vi "Begin.vi"(8 "error in":errorcluster) -> (0 "error out":errorcluster)   [LabVIEW 2014]
doc: "Called before other user functions, this VI is expected to open initial I/O refnums, load in file data, and do all program initialization. Notice that the <B>error out</B> terminal is simply used for data flow. Wiring it to other structures or subVIs ensures that this VI runs first."
uses:
  <vilib>/Rock Robotics/WPI/SafetyOutput/WPI_SafetyOutputConfigMenu.ctl
  Robot Global Data.vi
  <vilib>/Rock Robotics/WPI/DriverStation/WPI_DriverStationRobotMode2.ctl
  <vilib>/Rock Robotics/WPI/Joystick/WPI_JoystickDeviceEnum.ctl
  <vilib>/Rock Robotics/SystemInterfaces/DIO/FPGA_DIOPWMChannel.ctl
  <vilib>/Rock Robotics/Network Tables/SD Write String Array.vi
  <vilib>/Rock Robotics/WPI/RobotDrive/WPI_RobotDriveOpen4MotorWithTalon.vi
  <vilib>/Rock Robotics/WPI/MotorControl/WPI_MotorControlOpen Talon.vi
  <vilib>/Rock Robotics/WPI/Counter/WPI_CounterDigitalInputToDigitalSource.vi
  <vilib>/Rock Robotics/SystemInterfaces/DIO/FPGA_DIOChannel.ctl
  <vilib>/Rock Robotics/Network Tables/SD Write Number.vi
  <vilib>/Rock Robotics/SystemInterfaces/AI/FPGA_AIGyroChannel.ctl
  <vilib>/Rock Robotics/SystemInterfaces/AI/FPGA_AIChannel.ctl
panel:
  # "t"
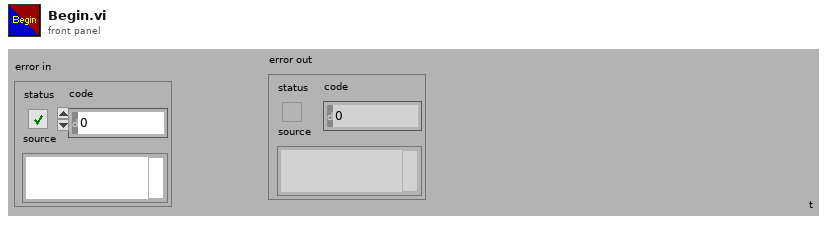
[diagram p1: front panel]
types:
  T1 = enum16{"Start", "Extending", "Lowering", "Grabbing", "Lifting", "Holding", "Placing", "Opening", "Dropping", "Score", "Exit", "Manual"}
  T2 = typedef "FPGA_DIOChannel.ctl" = enum8{"DIO 0", "DIO 1", "DIO 2", "DIO 3", "DIO 4", "DIO 5", "DIO 6", "DIO 7", "DIO 8", "DIO 9", "DIO MXP 0", "DIO MXP 1", "DIO MXP 2", "DIO MXP 3", "DIO MXP 4", "DIO MXP 5", "DIO MXP 6", "DIO MXP 7", "DIO MXP 8", "DIO MXP 9", "DIO MXP 10", "DIO MXP 11", "DIO MXP 12", "DIO MXP 13", "DIO MXP 14", "DIO MXP 15", "Invalid"}
  T3 = typedef "FPGA_AIChannel.ctl" = enum8{"AI 0", "AI 1", "AI 2", "AI 3", "AI MXP 0", "AI MXP 1", "AI MXP 2", "AI MXP 3", "Invalid"}
  T4 = typedef "FPGA_AIGyroChannel.ctl" = enum8{"AI 0", "AI 1", "Invalid"}
  T5 = typedef "FPGA_DIOPWMChannel.ctl" = enum8{"PWM 0", "PWM 1", "PWM 2", "PWM 3", "PWM 4", "PWM 5", "PWM 6", "PWM 7", "PWM 8", "PWM 9", "PWM MXP 0", "PWM MXP 1", "PWM MXP 2", "PWM MXP 3", "PWM MXP 4", "PWM MXP 5", "PWM MXP 6", "PWM MXP 7", "PWM MXP 8", "PWM MXP 9", "Invalid"}
  T6 = typedef "WPI_JoystickDeviceEnum.ctl" = enum16{"USB 0", "USB 1", "USB 2", "USB 3", "USB 4", "USB 5"}
  T7 = typedef "WPI_DriverStationRobotMode2.ctl" = enum16{"Autonomous Disabled", "Autonomous Enabled", "Teleop Disabled", "Teleop Enabled", "Disconnected", "Finish", "Test Disabled", "Test Enabled", "Emergency Stopped"}
  T8 = typedef "WPI_SafetyOutputConfigMenu.ctl" = enum16{"Enable", "Disable"}
  T9 = typedef "WPI_MotorControlDeviceRef.ctl" = cluster{"DeviceStatus":errorcluster, "Type":T10, "PWM":cluster{"Controller":T11, "PWM Channel":T5, "DeadBand":T12}, "CAN":cluster{"Device Number":u8, "Control Mode":T13, "Semaphore":T14, "Max Vout":dbl, "TalonSRX Control Mode":T15}, "Invert":bool, "TransformRef":T16, "InvTransformRef":T16}
  T10 = typedef "WPI_MotorControlType.ctl" = enum16{"PWM", "CAN", "CANTalonSRX"}
  T11 = typedef "FPGA_TypedefDigitalModule.ctl" = enum16{"Controller 1"}
  T12 = typedef "WPI_PWMDeadband.ctl" = cluster{"Name":string, "maxPositivePwm":i32, "minPositivePwm":i32, "centerPwm":i32, "maxNegativePwm":i32, "minNegativePwm":i32, "angularRange":u16}
  T13 = typedef "WPI_CANJaguar_ControlMode.ctl" = enum8{"Percent VBus", "Current", "Speed", "Position", "Voltage"}
  T14 = typedef "Semaphore RefNum" = refnum<k1>
  T15 = typedef "WPI_CANTalonSRX_APIControlMode.ctl" = enum8{"Percent VBus", "Speed", "Position", "Slave", "Unchanged / Invalid"}
  T16 = typedef "WPI_PWMTransform_ConPane.ctl" = refnum<vi>
  T17 = typedef "WPI_JoystickDevRef.ctl" = cluster{"Device":T6}
  T18 = typedef "WPI_RobotDriveDevRef.ctl" = cluster{"DevStatus":errorcluster, "Motors[]":T9[], "Square Inputs":bool, "Max Output":dbl}
  T19 = typedef "WPI_DigitalInputDevRef.ctl" = cluster{"DevStatus":errorcluster, "DIO Channel":T2, "Controller":T11}
  T20 = typedef "FPGA_CounterEncoderSourceConvertionLVSourceType.ctl" = cluster{"DevStatus":errorcluster, "AnalogTriggerMode?":bool, "DigitalMode":cluster{"Controller":T11, "DIO Channel":T21}, "AnalogTriggerMode":cluster{"AnalogTriggerIndex":T22, "OutputType":T23}}
  T21 = typedef "FPGA_DIODigitalSourceChannel.ctl" = enum8{"DIO 0", "DIO 1", "DIO 2", "DIO 3", "DIO 4", "DIO 5", "DIO 6", "DIO 7", "DIO 8", "DIO 9", "DIO MXP 0", "DIO MXP 1", "DIO MXP 2", "DIO MXP 3", "DIO MXP 4", "DIO MXP 5", "DIO MXP 6", "DIO MXP 7", "DIO MXP 8", "DIO MXP 9", "DIO MXP 10", "DIO MXP 11", "DIO MXP 12", "DIO MXP 13", "DIO MXP 14", "DIO MXP 15", "Disabled"}
  T22 = typedef "FPGA_AnalogTriggerIndex.ctl" = enum8{"Trig 0", "Trig 1", "Trig 2", "Trig 3", "Trig 4", "Trig 5", "Trig 6", "Trig 7", "Invalid"}
  T23 = typedef "FPGA_AnalogTriggerOutType.ctl" = enum16{"InWindow", "TriggerState", "Rising", "Falling"}
  T24 = typedef "WPI_EncoderDevRef.ctl" = cluster{"DevStatus":errorcluster, "EncoderIndex":T25, "CounterIndex":T26, "DistancePerCount":dbl, "Decoding Type":T27}
  T25 = typedef "FPGA_EncoderIdx.ctl" = enum8{"Enc 0", "Enc 1", "Enc 2", "Enc 3", "Enc 4", "Enc 5", "Enc 6", "Enc 7", "Invalid"}
  T26 = typedef "FPGA_CounterCtrSystemIndex.ctl" = enum8{"Ctr 0", "Ctr 1", "Ctr 2", "Ctr 3", "Ctr 4", "Ctr 5", "Ctr 6", "Ctr 7", "Invalid"}
  T27 = typedef "WPI_EncoderType.ctl" = enum16{"1x", "2x", "4x"}
  T28 = typedef "WPI_GyroDevRef.ctl" = cluster{"DevStatus":errorcluster, "Analog Module":T29, "Analog Channel":T3, "Offset":dbl, "Gain (VoltsPerDegree/Second)":dbl}
  T29 = typedef "FPGA_TypedefAnalogModule.ctl" = enum16{"Controller 1"}
  T30 = typedef "WPI_AnalogChannelDevRef.ctl" = cluster{"DevStatus":errorcluster, "Controller":T29, "Analog Channel":T3}
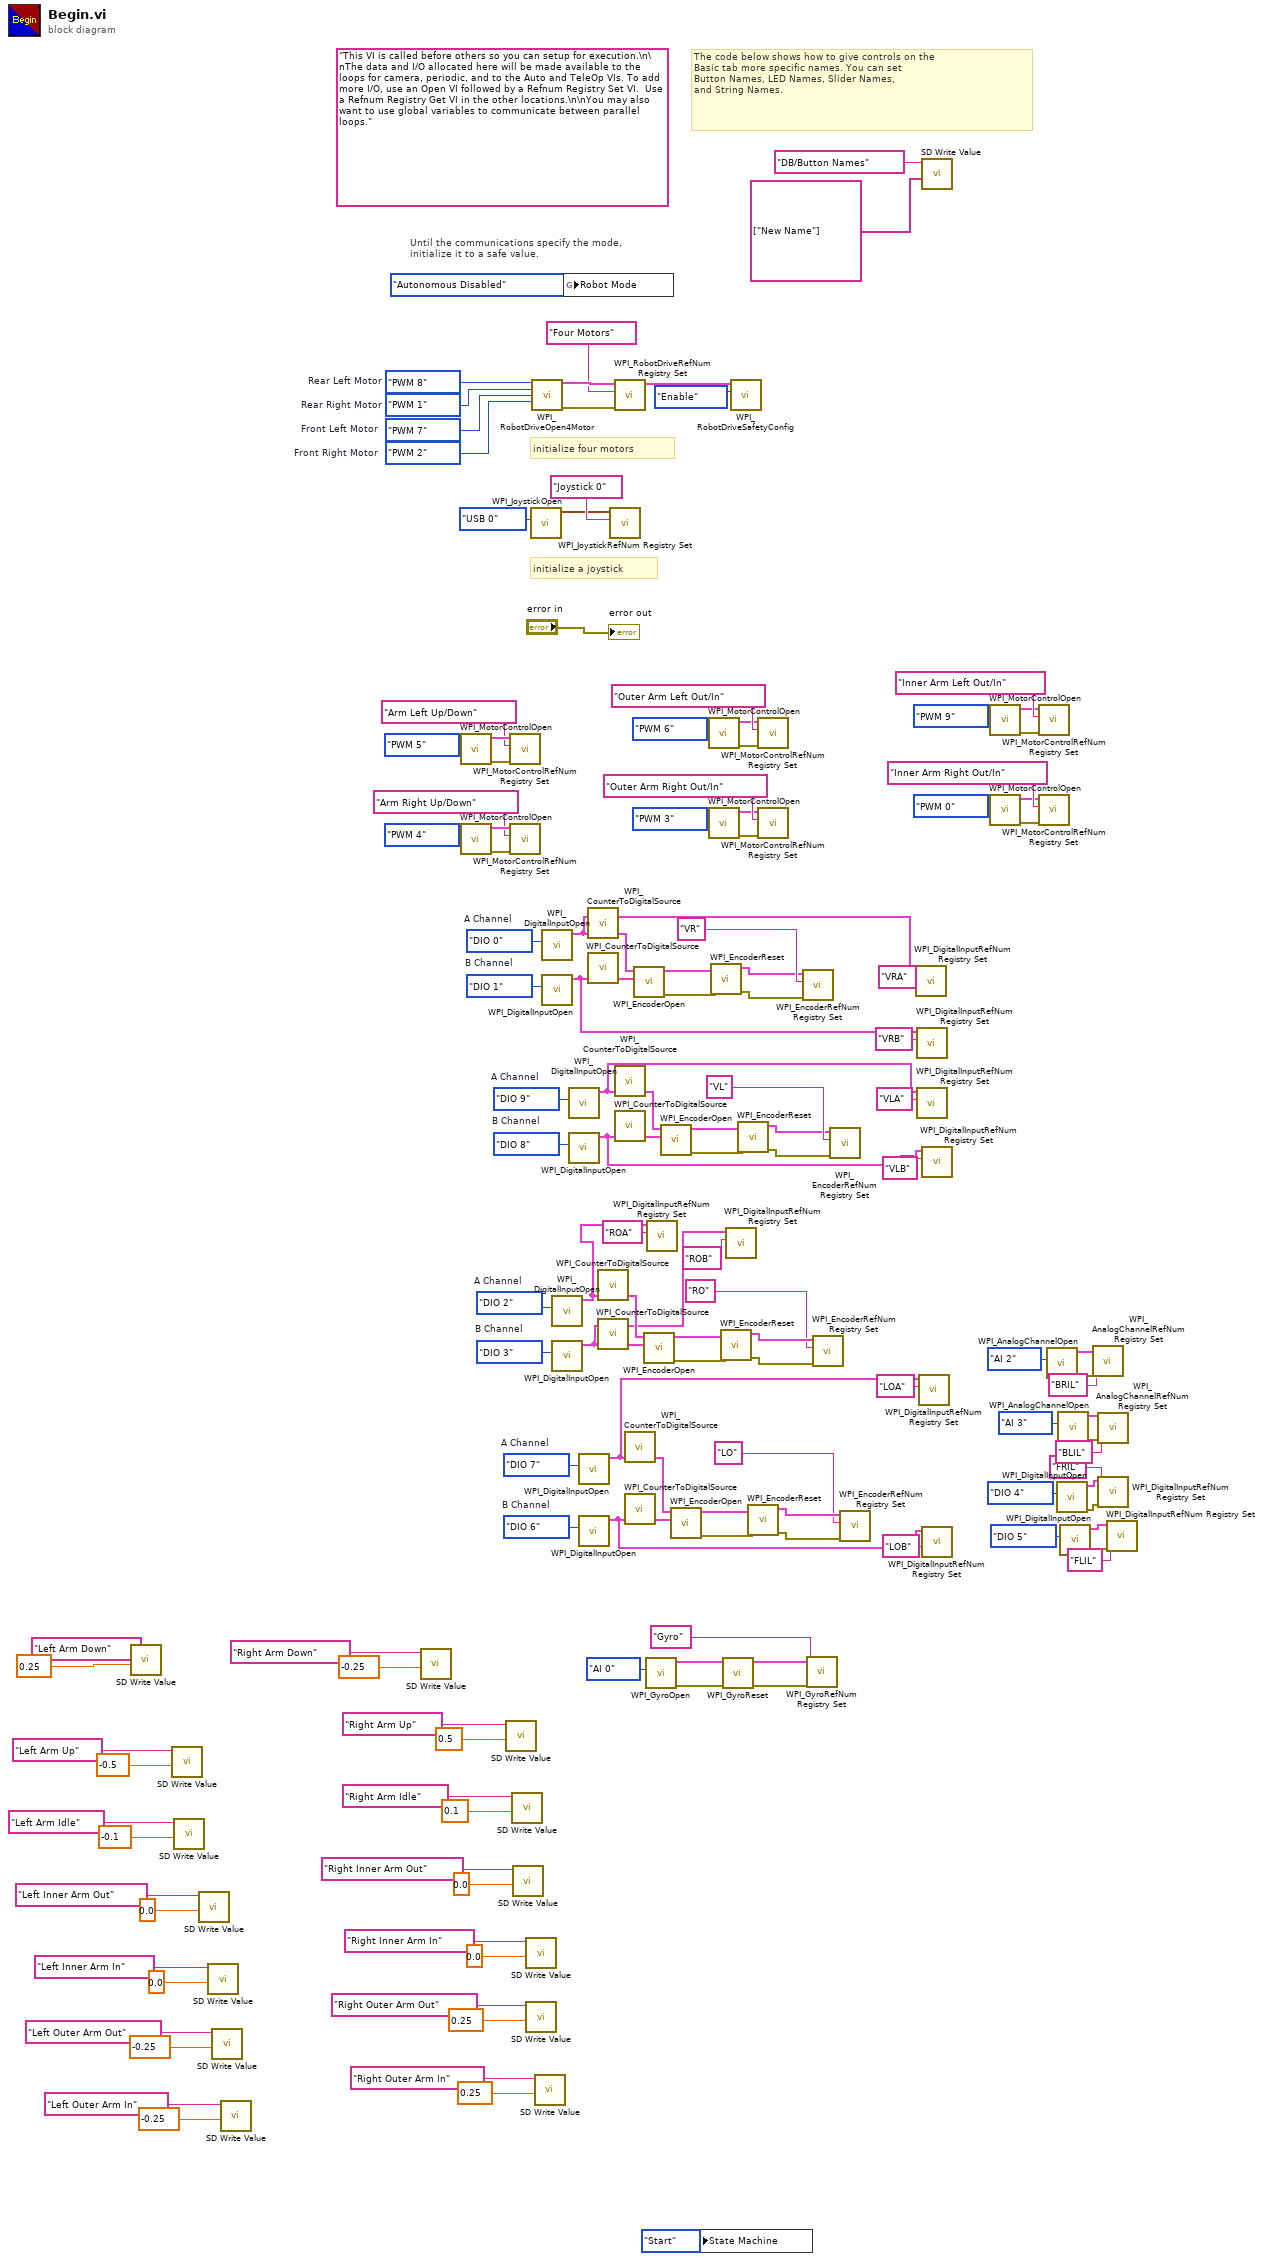
[diagram p0: block diagram]
diagram:
  w77 = FPGA_DIOChannel."DIO 6"  # B Channel
  w78 = FPGA_DIOChannel."DIO 7"  # A Channel
  w68 = FPGA_DIOChannel."DIO 3"  # B Channel
  w69 = FPGA_DIOChannel."DIO 2"  # A Channel
  w94 = FPGA_DIOChannel."DIO 8"  # B Channel
  w93 = FPGA_DIOChannel."DIO 9"  # A Channel
  w103 = FPGA_DIOChannel."DIO 1"  # B Channel
  w102 = FPGA_DIOChannel."DIO 0"  # A Channel
  w131 = FPGA_DIOPWMChannel."PWM 2"  # Front Right Motor
  w132 = FPGA_DIOPWMChannel."PWM 7"  # Front Left Motor
  w133 = FPGA_DIOPWMChannel."PWM 1"  # Rear Right Motor
  w134 = FPGA_DIOPWMChannel."PWM 8"  # Rear Left Motor
  (unwired) "This VI is called before others so you can setup for execution.\n\nThe data and I/O allocated here will be made available to the loops for camera, periodic, and to the Auto and TeleOp VIs. To add more I/O, use an Open VI followed by a Refnum Registry Set VI.  Use a Refnum Registry Get VI in the other locations.\n\nYou may also want to use global variables to communicate between parallel loops."
  # "The code below shows how to give controls on the\nBasic tab more specific names. You can set\nButton Names, LED Names, Slider Names,\nand String Names."
  # "initialize a joystick"
  # "Until the communications specify the mode,\ninitialize it to a safe value."
  # "initialize four motors"
  n1 = call-poly <vilib>:"SD Write Value.vi"("Numeric"=0.25, "Name"="Left Arm Down") -> ()  [unwired: 8 in, 2 out]
  n2 = call-poly <vilib>:"SD Write Value.vi"("Numeric"=-0.5, "Name"="Left Arm Up") -> ()  [unwired: 8 in, 2 out]
  n3 = call-poly <vilib>:"SD Write Value.vi"("Numeric"=-0.1, "Name"="Left Arm Idle") -> ()  [unwired: 8 in, 2 out]
  n4 = call-poly <vilib>:"SD Write Value.vi"("Numeric"=0.0, "Name"="Left Inner Arm Out") -> ()  [unwired: 8 in, 2 out]
  n5 = call-poly <vilib>:"SD Write Value.vi"("Numeric"=0.0, "Name"="Left Inner Arm In") -> ()  [unwired: 8 in, 2 out]
  n6 = call-poly <vilib>:"SD Write Value.vi"("Numeric"=-0.25, "Name"="Left Outer Arm Out") -> ()  [unwired: 8 in, 2 out]
  n7 = call-poly <vilib>:"SD Write Value.vi"("Numeric"=-0.25, "Name"="Left Outer Arm In") -> ()  [unwired: 8 in, 2 out]
  n8 = call-poly <vilib>:"SD Write Value.vi"("Numeric"=-0.25, "Name"="Right Arm Down") -> ()  [unwired: 8 in, 2 out]
  n9 = call-poly <vilib>:"WPI_MotorControlOpen.vi"("PWM Channel"=FPGA_DIOPWMChannel."PWM 5") -> ("error out"=w124:errorcluster, "MotorControlDeviceRef"=w125:T9)  [unwired: 9 in]
  n10 = call-poly <vilib>:"WPI_MotorControlOpen.vi"("PWM Channel"=FPGA_DIOPWMChannel."PWM 4") -> ("error out"=w126:errorcluster, "MotorControlDeviceRef"=w127:T9)  [unwired: 9 in]
  n11 = call-poly <vilib>:"SD Write Value.vi"("Numeric"=0.5, "Name"="Right Arm Up") -> ()  [unwired: 8 in, 2 out]
  n12 = call <vilib>:"WPI_MotorControlRefNum Registry Set.vi"("error in (no error)"=w124, "refnum name"="Arm Left Up/Down", "MotorControlDevRef"=w125) -> ()  [unwired: 7 in, 2 out]
  n13 = call <vilib>:"WPI_MotorControlRefNum Registry Set.vi"("error in (no error)"=w126, "refnum name"="Arm Right Up/Down", "MotorControlDevRef"=w127) -> ()  [unwired: 7 in, 2 out]
  n14 = call-poly <vilib>:"SD Write Value.vi"("Numeric"=0.1, "Name"="Right Arm Idle") -> ()  [unwired: 8 in, 2 out]
  n15 = call-poly <vilib>:"SD Write Value.vi"("Numeric"=0.0, "Name"="Right Inner Arm Out") -> ()  [unwired: 8 in, 2 out]
  n16 = call-poly <vilib>:"SD Write Value.vi"("Numeric"=0.0, "Name"="Right Inner Arm In") -> ()  [unwired: 8 in, 2 out]
  n17 = call-poly <vilib>:"SD Write Value.vi"("Numeric"=0.25, "Name"="Right Outer Arm Out") -> ()  [unwired: 8 in, 2 out]
  n18 = call <vilib>:"WPI_JoystickOpen.vi"("JoystickDevice"=WPI_JoystickDeviceEnum."USB 0") -> ("JoystickDevRef"=w136:T17)  [unwired: 10 in]
  n19 = call-poly <vilib>:"WPI_RobotDriveOpen4Motor.vi"("Rear Left Motor"=w134, "Rear Right Motor"=w133, "Front Left Motor"=w132, "Front Right Motor"=w131) -> ("RobotDriveDevRef"=w143:T18, "error out"=w141:errorcluster)  [unwired: 10 in]
  n20 = call-poly <vilib>:"SD Write Value.vi"("Numeric"=0.25, "Name"="Right Outer Arm In") -> ()  [unwired: 8 in, 2 out]
  n21 = call <vilib>:"WPI_DigitalInputOpen.vi"("DIO Channel"=w102) -> ("DigitalInputDevRef"=w63:T19)  [unwired: 2 in, 8 out]
  n22 = call <vilib>:"WPI_DigitalInputOpen.vi"("DIO Channel"=w103) -> ("DigitalInputDevRef"=w61:T19)  [unwired: 2 in, 8 out]
  n23 = call <vilib>:"WPI_DigitalInputOpen.vi"("DIO Channel"=w69) -> ("DigitalInputDevRef"=w67:T19)  [unwired: 2 in, 8 out]
  n24 = call <vilib>:"WPI_DigitalInputOpen.vi"("DIO Channel"=w68) -> ("DigitalInputDevRef"=w66:T19)  [unwired: 2 in, 8 out]
  n25 = global write "Robot Global Data.vi" "Robot Mode"(WPI_DriverStationRobotMode2."Autonomous Disabled" ("Robot Mode")) -> ()
  n26 = call <vilib>:"WPI_DigitalInputOpen.vi"("DIO Channel"=w93) -> ("DigitalInputDevRef"=w62:T19)  [unwired: 2 in, 8 out]
  n27 = call <vilib>:"WPI_DigitalInputOpen.vi"("DIO Channel"=w94) -> ("DigitalInputDevRef"=w60:T19)  [unwired: 2 in, 8 out]
  n28 = call <vilib>:"WPI_DigitalInputOpen.vi"("DIO Channel"=w78) -> ("DigitalInputDevRef"=w65:T19)  [unwired: 2 in, 8 out]
  n29 = call <vilib>:"WPI_DigitalInputOpen.vi"("DIO Channel"=w77) -> ("DigitalInputDevRef"=w64:T19)  [unwired: 2 in, 8 out]
  n30 = call-poly <vilib>:"WPI_CounterToDigitalSource.vi"("DigitalInputDevRef"=w63) -> ("Digital Source"=w100:T20)  [unwired: 6 out]
  n31 = call-poly <vilib>:"WPI_CounterToDigitalSource.vi"("DigitalInputDevRef"=w61) -> ("Digital Source"=w101:T20)  [unwired: 6 out]
  n32 = call-poly <vilib>:"WPI_CounterToDigitalSource.vi"("DigitalInputDevRef"=w67) -> ("Digital Source"=w71:T20)  [unwired: 6 out]
  n33 = call-poly <vilib>:"WPI_CounterToDigitalSource.vi"("DigitalInputDevRef"=w66) -> ("Digital Source"=w70:T20)  [unwired: 6 out]
  n34 = call <vilib>:"WPI_JoystickRefNum Registry Set.vi"("refnum name"="Joystick 0", "JoystickDevRef"=w136) -> ()  [unwired: 8 in, 2 out]
  n35 = call <vilib>:"WPI_RobotDriveRefNum Registry Set.vi"("error in (no error)"=w141, "refnum name"="Four Motors", "RobotDriveDevRef"=w143) -> ("RobotDriveDevRef"=w140:T18)  [unwired: 8 out]
  n36 = call-poly <vilib>:"WPI_CounterToDigitalSource.vi"("DigitalInputDevRef"=w62) -> ("Digital Source"=w91:T20)  [unwired: 6 out]
  n37 = call-poly <vilib>:"WPI_CounterToDigitalSource.vi"("DigitalInputDevRef"=w60) -> ("Digital Source"=w92:T20)  [unwired: 6 out]
  n38 = call-poly <vilib>:"WPI_CounterToDigitalSource.vi"("DigitalInputDevRef"=w65) -> ("Digital Source"=w80:T20)  [unwired: 6 out]
  n39 = call-poly <vilib>:"WPI_CounterToDigitalSource.vi"("DigitalInputDevRef"=w64) -> ("Digital Source"=w79:T20)  [unwired: 6 out]
  n40 = call <vilib>:"WPI_EncoderOpen.vi"("BSource"=w101, "ASource"=w100) -> ("error out"=w97:errorcluster, "EncoderDevRef"=w98:T24)  [unwired: 6 in, 2 out]
  n41 = call <vilib>:"WPI_EncoderOpen.vi"("BSource"=w70, "ASource"=w71) -> ("error out"=w74:errorcluster, "EncoderDevRef"=w73:T24)  [unwired: 6 in, 2 out]
  n42 = call <vilib>:"WPI_GyroOpen.vi"("Analog Channel"=FPGA_AIGyroChannel."AI 0") -> ("error out"=w18:errorcluster, "GyroDevRef"=w21:T28)  [unwired: 8 in, 1 out]
  n43 = call <vilib>:"WPI_DigitalInputRefNum Registry Set.vi"("refnum name"="ROA", "DigitalInputDevRef"=w67) -> ()  [unwired: 8 in, 2 out]
  n44 = call <vilib>:"WPI_EncoderOpen.vi"("BSource"=w92, "ASource"=w91) -> ("error out"=w88:errorcluster, "EncoderDevRef"=w89:T24)  [unwired: 6 in, 2 out]
  n45 = call <vilib>:"WPI_EncoderOpen.vi"("BSource"=w79, "ASource"=w80) -> ("error out"=w83:errorcluster, "EncoderDevRef"=w82:T24)  [unwired: 6 in, 2 out]
  n46 = global write "Robot Global Data.vi" "State Machine"(T1."Start" ("State Machine")) -> ()
  n47 = call-poly <vilib>:"WPI_MotorControlOpen.vi"("PWM Channel"=FPGA_DIOPWMChannel."PWM 6") -> ("error out"=w115:errorcluster, "MotorControlDeviceRef"=w114:T9)  [unwired: 9 in]
  n48 = call-poly <vilib>:"WPI_MotorControlOpen.vi"("PWM Channel"=FPGA_DIOPWMChannel."PWM 3") -> ("error out"=w113:errorcluster, "MotorControlDeviceRef"=w112:T9)  [unwired: 9 in]
  n49 = call <vilib>:"WPI_EncoderReset.vi"("error in (no error)"=w97, "EncoderDevRef"=w98) -> ("error out"=w95:errorcluster, "EncoderDevRef"=w96:T24)  [unwired: 8 in]
  n50 = call <vilib>:"WPI_EncoderReset.vi"("error in (no error)"=w74, "EncoderDevRef"=w73) -> ("error out"=w76:errorcluster, "EncoderDevRef"=w75:T24)  [unwired: 8 in]
  n51 = call <vilib>:"WPI_GyroReset.vi"("error in (no error)"=w18, "GyroDevRef"=w21) -> ("error out"=w19:errorcluster, "GyroDevRef"=w20:T28)  [unwired: 8 in]
  n52 = call <vilib>:"WPI_DigitalInputRefNum Registry Set.vi"("refnum name"="ROB", "DigitalInputDevRef"=w66) -> ()  [unwired: 8 in, 2 out]
  n53 = call <vilib>:"WPI_RobotDriveSafetyConfig.vi"("mode"=WPI_SafetyOutputConfigMenu."Enable", "RobotDriveDevRef"=w140) -> ()  [unwired: 8 in, 2 out]
  n54 = call <vilib>:"WPI_EncoderReset.vi"("error in (no error)"=w88, "EncoderDevRef"=w89) -> ("error out"=w86:errorcluster, "EncoderDevRef"=w87:T24)  [unwired: 8 in]
  n55 = call <vilib>:"WPI_EncoderReset.vi"("error in (no error)"=w83, "EncoderDevRef"=w82) -> ("error out"=w85:errorcluster, "EncoderDevRef"=w84:T24)  [unwired: 8 in]
  n56 = call <vilib>:"WPI_MotorControlRefNum Registry Set.vi"("error in (no error)"=w115, "refnum name"="Outer Arm Left Out/In", "MotorControlDevRef"=w114) -> ()  [unwired: 7 in, 2 out]
  n57 = call <vilib>:"WPI_MotorControlRefNum Registry Set.vi"("error in (no error)"=w113, "refnum name"="Outer Arm Right Out/In", "MotorControlDevRef"=w112) -> ()  [unwired: 7 in, 2 out]
  n58 = call <vilib>:"WPI_EncoderRefNum Registry Set.vi"("error in (no error)"=w95, "refnum name"="VR", "EncoderDevRef"=w96) -> ()  [unwired: 7 in, 2 out]
  n59 = call <vilib>:"WPI_GyroRefNum Registry Set.vi"("error in (no error)"=w19, "refnum name"="Gyro", "GyroDevRef"=w20) -> ()  [unwired: 7 in, 2 out]
  n60 = call <vilib>:"WPI_EncoderRefNum Registry Set.vi"("error in (no error)"=w76, "refnum name"="RO", "EncoderDevRef"=w75) -> ()  [unwired: 7 in, 2 out]
  n61 = call <vilib>:"WPI_EncoderRefNum Registry Set.vi"("error in (no error)"=w86, "refnum name"="VL", "EncoderDevRef"=w87) -> ()  [unwired: 7 in, 2 out]
  n62 = call <vilib>:"WPI_EncoderRefNum Registry Set.vi"("error in (no error)"=w85, "refnum name"="LO", "EncoderDevRef"=w84) -> ()  [unwired: 7 in, 2 out]
  n63 = call <vilib>:"WPI_DigitalInputRefNum Registry Set.vi"("refnum name"="VRA", "DigitalInputDevRef"=w63) -> ()  [unwired: 8 in, 2 out]
  n64 = call <vilib>:"WPI_DigitalInputRefNum Registry Set.vi"("refnum name"="VRB", "DigitalInputDevRef"=w61) -> ()  [unwired: 8 in, 2 out]
  n65 = call <vilib>:"WPI_DigitalInputRefNum Registry Set.vi"("refnum name"="VLA", "DigitalInputDevRef"=w62) -> ()  [unwired: 8 in, 2 out]
  n66 = call <vilib>:"WPI_DigitalInputRefNum Registry Set.vi"("refnum name"="LOA", "DigitalInputDevRef"=w65) -> ()  [unwired: 8 in, 2 out]
  n67 = call-poly <vilib>:"SD Write Value.vi"("String Array"=string[] ["New Name"], "Name"="DB/Button Names") -> ()  [unwired: 8 in, 2 out]
  n68 = call <vilib>:"WPI_DigitalInputRefNum Registry Set.vi"("refnum name"="VLB", "DigitalInputDevRef"=w60) -> ()  [unwired: 8 in, 2 out]
  n69 = call <vilib>:"WPI_DigitalInputRefNum Registry Set.vi"("refnum name"="LOB", "DigitalInputDevRef"=w64) -> ()  [unwired: 8 in, 2 out]
  n70 = call-poly <vilib>:"WPI_MotorControlOpen.vi"("PWM Channel"=FPGA_DIOPWMChannel."PWM 9") -> ("error out"=w107:errorcluster, "MotorControlDeviceRef"=w106:T9)  [unwired: 9 in]
  n71 = call-poly <vilib>:"WPI_MotorControlOpen.vi"("PWM Channel"=FPGA_DIOPWMChannel."PWM 0") -> ("error out"=w105:errorcluster, "MotorControlDeviceRef"=w104:T9)  [unwired: 9 in]
  n72 = call <vilib>:"WPI_MotorControlRefNum Registry Set.vi"("error in (no error)"=w107, "refnum name"="Inner Arm Left Out/In", "MotorControlDevRef"=w106) -> ()  [unwired: 7 in, 2 out]
  n73 = call <vilib>:"WPI_MotorControlRefNum Registry Set.vi"("error in (no error)"=w105, "refnum name"="Inner Arm Right Out/In", "MotorControlDevRef"=w104) -> ()  [unwired: 7 in, 2 out]
  n74 = call <vilib>:"WPI_AnalogChannelOpen.vi"("Analog Channel"=FPGA_AIChannel."AI 2") -> ("error out"=w17:errorcluster, "AIDeviceRef"=w16:T30)  [unwired: 9 in]
  n75 = call <vilib>:"WPI_DigitalInputOpen.vi"("DIO Channel"=FPGA_DIOChannel."DIO 4") -> ("error out"=w7:errorcluster, "DigitalInputDevRef"=w6:T19)  [unwired: 9 in]
  n76 = call <vilib>:"WPI_AnalogChannelOpen.vi"("Analog Channel"=FPGA_AIChannel."AI 3") -> ("error out"=w15:errorcluster, "AIDeviceRef"=w14:T30)  [unwired: 9 in]
  n77 = call <vilib>:"WPI_DigitalInputOpen.vi"("DIO Channel"=FPGA_DIOChannel."DIO 5") -> ("error out"=w4:errorcluster, "DigitalInputDevRef"=w5:T19)  [unwired: 9 in]
  n78 = call <vilib>:"WPI_AnalogChannelRefNum Registry Set.vi"("error in (no error)"=w17, "refnum name"="BRIL", "AIDeviceRef"=w16) -> ()  [unwired: 7 in, 2 out]
  n79 = call <vilib>:"WPI_AnalogChannelRefNum Registry Set.vi"("error in (no error)"=w15, "refnum name"="BLIL", "AIDeviceRef"=w14) -> ()  [unwired: 7 in, 2 out]
  n80 = call <vilib>:"WPI_DigitalInputRefNum Registry Set.vi"("error in (no error)"=w7, "refnum name"="FRIL", "DigitalInputDevRef"=w6) -> ()  [unwired: 7 in, 2 out]
  n81 = call <vilib>:"WPI_DigitalInputRefNum Registry Set.vi"("error in (no error)"=w4, "refnum name"="FLIL", "DigitalInputDevRef"=w5) -> ()  [unwired: 7 in, 2 out]
  "error out" <- "error in"
